vi "arcade_drive.vi"(9 "velocity_rat":dbl, 10 "turn":dbl, 11 "mpower":cluster{"left":dbl, "right":dbl}) -> (3 "mpower":cluster{"left":dbl, "right":dbl})   [LabVIEW 2014]
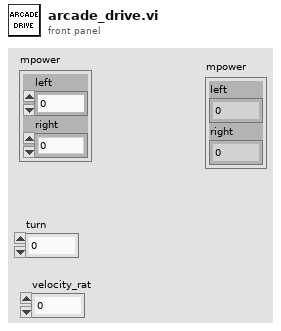
[diagram p1: front panel]
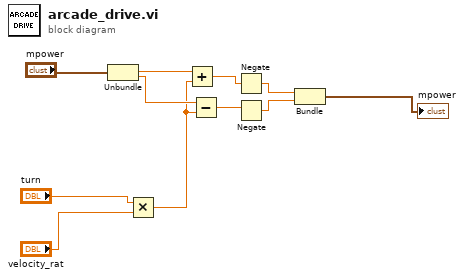
[diagram p0: block diagram]
diagram:
  n1 = Unbundle("mpower") -> ("left"=w10:dbl, "right"=w9:dbl)
  n2 = Multiply(x="turn", y="velocity_rat") -> (x*y=w7:dbl)
  n3 = Add(x=w10, y=w7) -> (x+y=w4:dbl)
  n4 = Subtract(x=w9, y=w7) -> (x-y=w2:dbl)
  n5 = Negate(x=w4) -> (-x=w3:dbl)
  n6 = Negate(x=w2) -> (-x=w1:dbl)
  n7 = Bundle(w3, w1) -> (→"mpower":cluster{dbl, dbl})  [unwired: 1 in]
